vi "Stringfunctionsv15.vi"() -> ()   [LabVIEW 2015]
uses:
  <vilib>/regexp/Match Regular Expression.xnode
panel:
  out "error out":errorcluster
  out "resulting string":string
  in  "Val 2":dbl
  in  "Val1":dbl
  in  "String 6":string
  in  "regular expression":string
  out "after match String 6":string
  out "whole match String 6":string
  out "before match String 6":string
  out "output 3":i32
  out "output 2":string
  out "output 1":cdb
  out "remaining string":string
  in  "format string":string
  in  "initial scan location":u32
  in  "String 5":string
  out "Array --> Path":path
  out "Path --> String":string
  out "Relative path?":bool
  out "Array of strings (Path)":string[](array[string])
  in  "Path":path
  in  "stop":bool
  out "number of replacements":i32
  out "result string 4":string
  in  "replace all? (F)":bool
  in  "Empezar en":i32
  in  "replace string (\"\")":string
  in  "search string":string
  in  "String 4":string
  out "reemplazo de string 3":string
  out "elemento reemplazado":string
  in  "substring (\"\")":string
  in  "offset (0)":i32
  in  "length (len. of substring)":i32
  out "trimmed of string 3":string
  in  "String 3":string
  in  "Largor":i32
  in  "Subset comienzo":i32
  out "String 2 subset":string
  out "String 1 + String 2":string
  in  "String 2":string
  out "String 1 length":i32
  in  "String 1":string
  # "Observe que las constantes\nen el block diagram \ndeterminan lo que se hace."
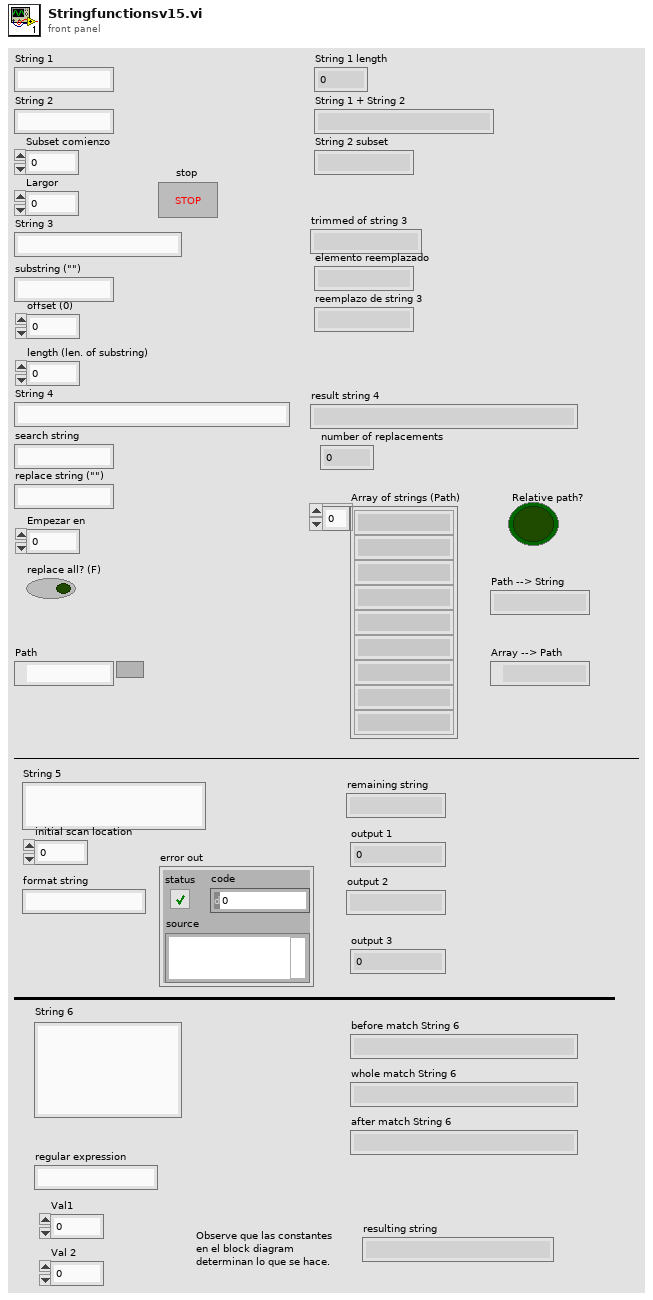
[diagram p1: front panel]
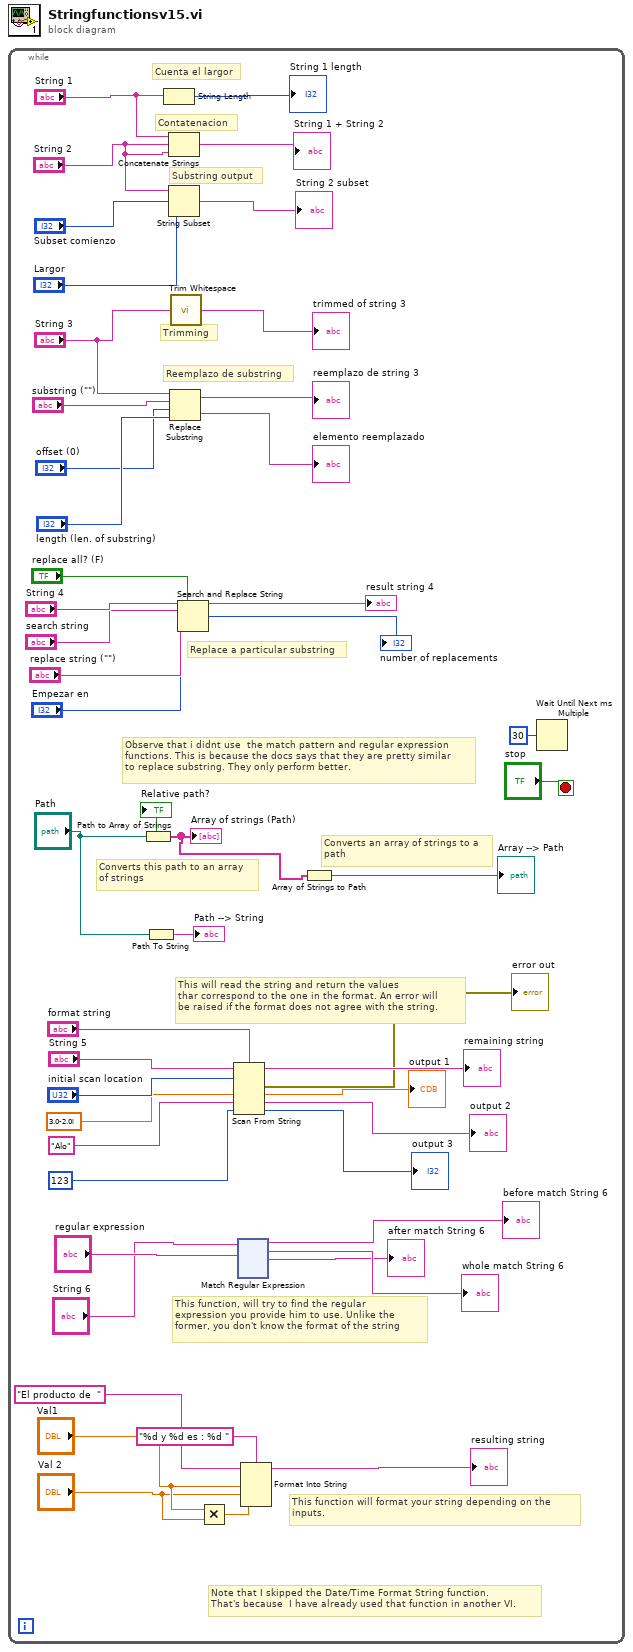
[diagram p0: block diagram]
diagram:
  n1 = while {
    stop <- "stop" stop-if-true
    # "Note that I skipped the Date/Time Format String function.\nThat's because  I have already used that function in another VI."
    # "This function will format your string depending on the\ninputs."
    # "This function, will try to find the regular\nexpression you provide him to use. Unlike the\nformer, you don't know the format of the string"
    # "This will read the string and return the values \nthar correspond to the one in the format. An error will \nbe raised if the format does not agree with the string."
    # "Converts an array of strings to a\npath"
    # "Converts this path to an array \nof strings"
    # "Observe that i didnt use  the match pattern and regular expression\nfunctions. This is because the docs says that they are pretty similar\nto replace substring. They only perform better."
    # "Replace a particular substring"
    # "Reemplazo de substring"
    # "Trimming"
    # "Substring output"
    # "Contatenacion"
    # "Cuenta el largor"
    n2 = Path to Array of Strings(0:"Path") -> (1:→"Relative path?":bool, 2:w24:string[])
    "Array of strings (Path)" <- w24
    n3 = Path To String(path="Path") -> (string=→"Path --> String":string)
    n4 = String Length(string="String 1") -> (length=→"String 1 length":i32)
    n5 = Concatenate Strings("String 1", "String 2", "String 2") -> (→"String 1 + String 2":string)
    n6 = String Subset(string="String 2", offset (0)="Subset comienzo", length (rest)="Largor") -> (substring=→"String 2 subset":string)
    n7 = Replace Substring(2:"length (len. of substring)", 3:"offset (0)", 4:"substring (\"\")", 5:"String 3") -> (0:→"elemento reemplazado":string, 1:→"reemplazo de string 3":string)
    n8 = call <vilib>:"Trim Whitespace.vi"("string"="String 3") -> ("trimmed string"=→"trimmed of string 3":string)  [unwired: 1 in]
    n9 = Search and Replace String(replace all?="replace all? (F)", input string="String 4", search string="search string", replace string="replace string (\"\")", offset="Empezar en") -> (result string=→"result string 4":string, number of replacements=→"number of replacements":i32)  [unwired: 3 in, 2 out]
    n10 = Multiply(x="Val1", y="Val 2") -> (x*y=w5:dbl)
    n11 = Scan From String(format string="format string", input string="String 5", initial scan location="initial scan location", default 1=cdb 3.0-2.0i ("default value 1"), default 2="Alo", default 3=123) -> (remaining string=→"remaining string":string, error out=→"error out":errorcluster, output 1=→"output 1":cdb, output 2=→"output 2":string, output 3=→"output 3":i32)  [unwired: 1 in, 1 out]
    n12 = xnode "Match Regular Expression"("input string"="String 6", "regular expression"="regular expression") -> ("before match"=→"before match String 6":string, "whole match"=→"whole match String 6":string, "after match"=→"after match String 6":string)  [unwired: 4 in, 2 out]
    n13 = Format Into String(format string="%d y %d es : %d ", initial string="El producto de  ", "Val1", "Val 2", w5) -> (resulting string=→"resulting string":string)  [unwired: 1 in, 1 out]
    n14 = Array of Strings to Path(0:w24) -> (2:→"Array --> Path":path)  [unwired: 1 in]
    n15 = Wait Until Next ms Multiple(millisecond multiple=u32 30) -> ()  [unwired: 1 out]
  }
